vi "update table.vi"(8 "error in (no error)":errorcluster, 10 "Table in":refnum<vi>, 11 "State":T1={"logTable"=refnum, "max items"=500, "displaydata"=[], "data"=[], "Auto Scroll"=TRUE, "current item"=500, "col headers"=[], "Add to Top"=TRUE, "Auto resize"=TRUE, "col size"=[], "filters"=[], "color cells"=[]}) -> (0 "error out":errorcluster, 2 "Table out":refnum<vi>, 3 "State (dup)":T1={"logTable"=refnum, "max items"=500, "displaydata"=[], "data"=[], "Auto Scroll"=TRUE, "current item"=500, "col headers"=[], "Add to Top"=TRUE, "Auto resize"=TRUE, "col size"=[], "filters"=[], "color cells"=[]})   [LabVIEW 2017, in "UI-DisplayTable(dev).xctl"]
uses:
  UI-DisplayTable(dev).xctl
  State.ctl
  DEF-Filter.ctl
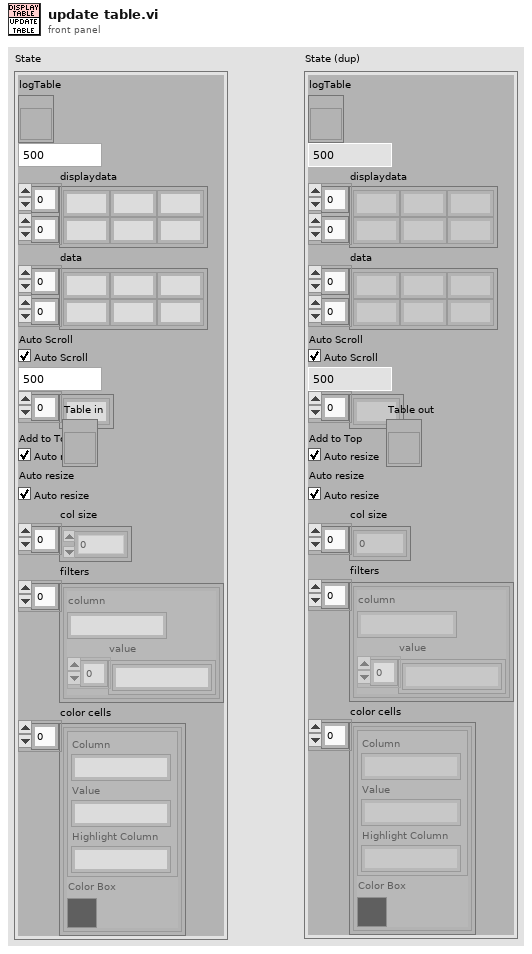
[diagram p1: front panel]
types:
  T1 = typedef "UI-DisplayTable(dev).xctl/State.ctl" = cluster{"logTable":refnum<vi>, "max items":i32, "displaydata":string[][], "data":string[][], "Auto Scroll":bool, "current item":i32, "col headers":string[], "Add to Top":bool, "Auto resize":bool, "col size":i32[], "filters":T2[], "color cells":cluster{"color cell":cluster{"Column":string, "Value":string, "Highlight Column":string}, "Color Box":u32}[]}
  T2 = typedef "UI-DisplayTable(dev).xctl/DEF-Filter.ctl" = cluster{"column":string, "value":string[]}
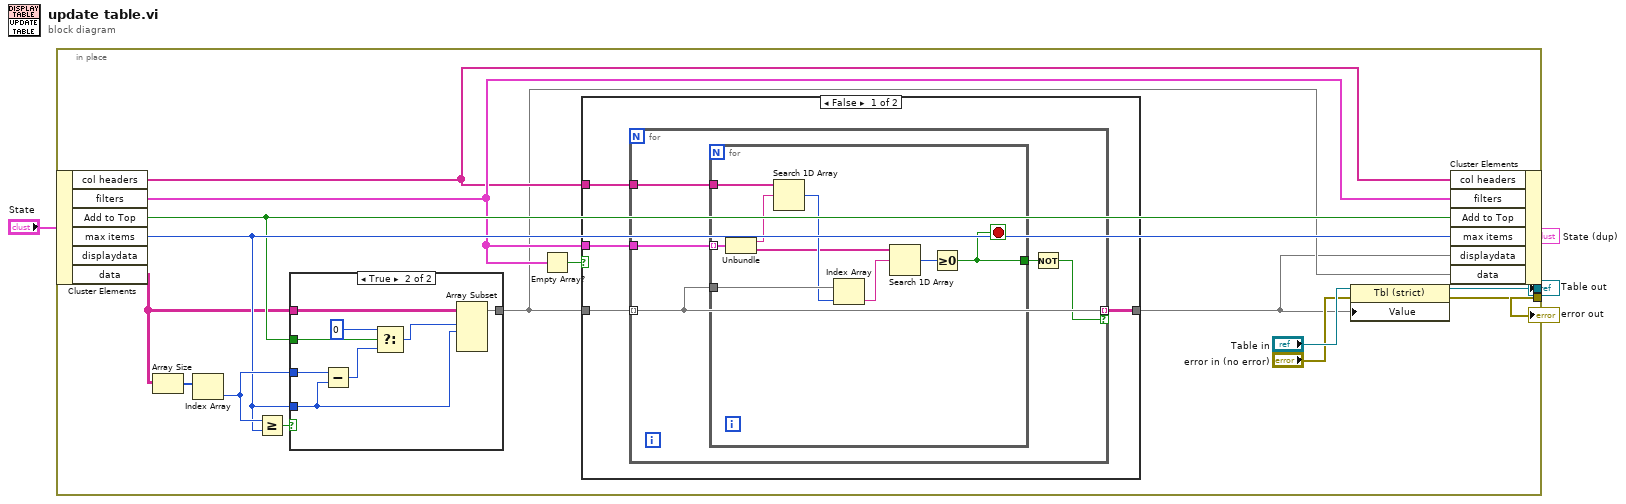
[diagram p0: block diagram]
diagram:
  n1 = in-place {
    in-place-border: [w15] -> w4
    in-place-border: [w13] -> w3
    n2 = in-place-cluster #1("State") -> ("col headers"=w8:string[], "filters"=w9:T2[], "Add to Top"=w11:bool, "max items"=w12:i32, "data"=w5:string[][])  [unwired: 1 out]
    n3 = Array Size(array=w5) -> (size(s)=w19:i32[])
    n4 = Index Array(array=w19) -> (element=w17:i32)  [unwired: 1 in]
    n5 = Greater Or Equal?(x=w17, y=w12) -> (x >= y?=w18:bool)
    n6 = case shown="True" w18 {
      tunnel: w5 -> [w39 w47]
      tunnel: w12 -> [_ w44]
      tunnel: w17 -> [_ w46]
      tunnel: [w39 w45] -> w7
      tunnel: w11 -> [_ w43]
      frame False {
      }
      frame True {
        n7 = Subtract(x=w46, y=w44) -> (x-y=w40:i32)
        n8 = Select(t=0, s=w43, f=w40) -> (s? t:f=w42:i32)
        n9 = Array Subset(array=w47, index (row)=w42, length (row)=w44) -> (w45:string[][])  [unwired: 2 in]
      }
    }
    n10 = Empty Array?(array=w9) -> (empty?=w10:bool)
    n11 = case shown="False" w10 {
      tunnel: [w22 w38] -> w6
      tunnel: w7 -> [w23 w38]
      tunnel: w9 -> [w21 _]
      tunnel: w8 -> [w20 _]
      frame False {
        n12 = for {
          tunnel: w23 -> [w26] mode=indexing
          tunnel: [w26] -> w22 mode=indexing if=w24
          tunnel: w21 -> [w27]
          tunnel: w20 -> [w28]
          n13 = for {
            tunnel: w28 -> [w37]
            tunnel: w27 -> [w36] mode=indexing
            tunnel: w26 -> [w34]
            tunnel: [w29] -> w25
            stop <- w29 stop-if-true
            n14 = Unbundle(w36) -> ("column"=w35:string, "value"=w31:string[])
            n15 = Search 1D Array(1D array=w37, element=w35) -> (index of element=w33:i32)  [unwired: 1 in]
            n16 = Index Array(array=w34, index=w33) -> (element=w32:string)
            n17 = Search 1D Array(1D array=w31, element=w32) -> (index of element=w30:i32)  [unwired: 1 in]
            n18 = Greater Or Equal To 0?(x=w30) -> (x >= 0?=w29:bool)
          }
          n19 = Not(x=w25) -> (.not. x?=w24:bool)
        }
      }
      frame True {
      }
    }
    n20 = property on="Property Node" class="Tbl (strict)"(reference="Table in", error in="error in (no error)", "Value"=w6) -> (reference out=w15:refnum<vi>, error out=w13:errorcluster)
    n21 = in-place-cluster #1("col headers"=w8, "filters"=w9, "Add to Top"=w11, "max items"=w12, "displaydata"=w6, "data"=w7) -> (→"State (dup)":T1)
  }
  "error out" <- w3
  "Table out" <- w4
